vi "Samsung Test Bench.vi"() -> ()   [LabVIEW 2014]
uses:
  Controls/NamedError.ctl
  Controls/ES String Data.ctl
  Controls/ES String Array.ctl
  Controls/StringSelector.ctl
  Controls/ES System Data.ctl
  Controls/Gen Data.ctl
panel:
  out "Generator Fault String":string
  out "Generator Data":T1 {"Alarms" format="%04x"}
  out "PDP Control Error":T2
  in  "PDP Contact On":bool
  in  "Reset Samsung":bool
  in  "Clear Error":bool
  in  "Generator On":bool
  out "Generator Error":T2
  out "Voltage 2":sgl format="%3.0f V"
  out "Voltage 1":sgl format="%3.0f V"
  in  "Contactor 2":bool
  in  "Contactor 1":bool
  out "Battery System Data":T3={"Voltage"=0.0, "Current"=0.0, "SOC Avg"=0.0, "Faults"=0, "Alarms"=0, "# Strings"=0, "Max Temp"=0, "Min Temp"=0, "Max Cell Voltage"=0.0, "Min Cell Voltage"=0.0, "Energy Capacity"=0.0, "Energy Remaining"=0.0, "SOC Min"=0.0, "SOC Max"=0.0, "ES Fault"=FALSE, "String Select"=enum."3 Strings", "ES Com Fault"=FALSE, "SOH Avg"=0.0}
  out "Battery Rack Data":T5
  out "Battery Error":T2
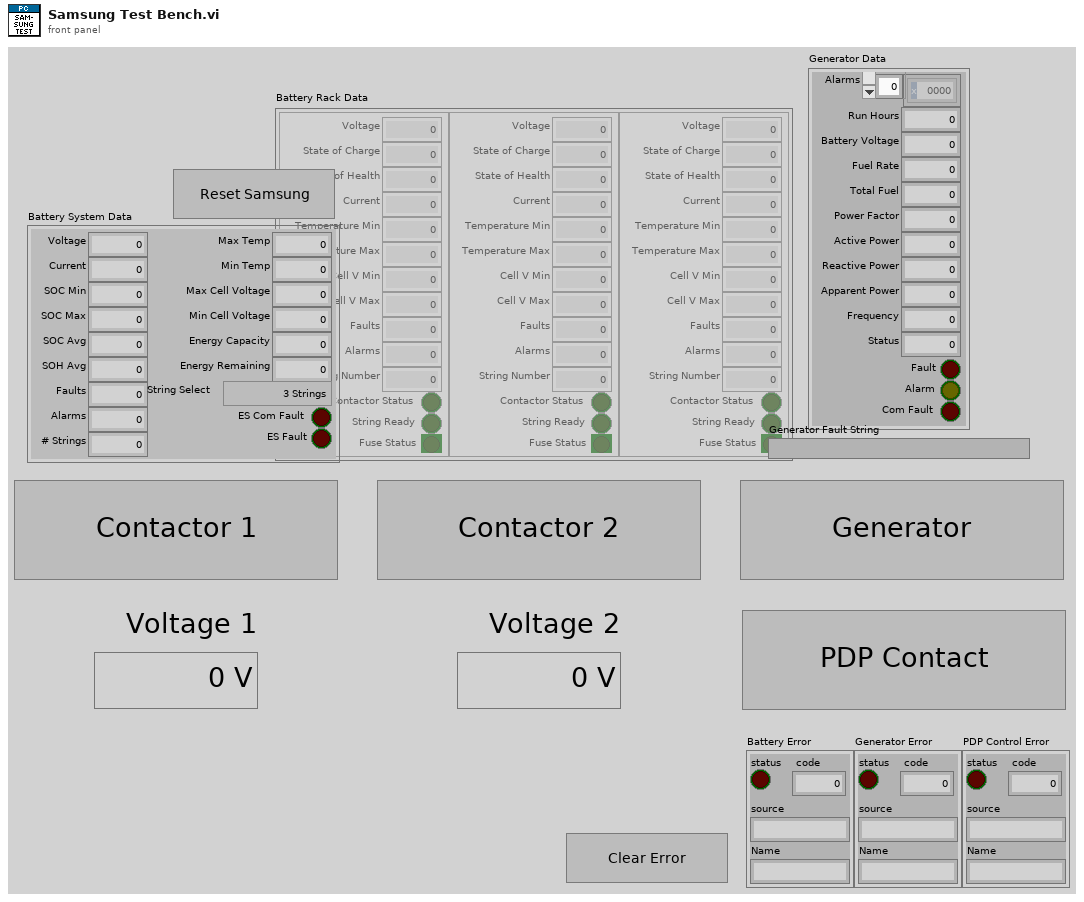
[diagram p1: front panel]
types:
  T1 = typedef "Gen Data.ctl" = cluster{"Alarms":i16[], "Run Hours":dbl, "Battery Voltage":dbl, "Fuel Rate":dbl, "Total Fuel":dbl, "Power Factor":dbl, "Active Power":dbl, "Reactive Power":dbl, "Apparent Power":dbl, "Frequency":dbl, "Status":u16, "Fault":bool, "Alarm":bool, "Com Fault":bool}
  T2 = typedef "NamedError.ctl" = cluster{"status":bool, "code":i32, "source":string, "Name":string}
  T3 = typedef "ES System Data.ctl" = cluster{"Voltage":sgl, "Current":sgl, "SOC Avg":sgl, "Faults":u16, "Alarms":u16, "# Strings":u16, "Max Temp":i16, "Min Temp":i16, "Max Cell Voltage":sgl, "Min Cell Voltage":sgl, "Energy Capacity":sgl, "Energy Remaining":sgl, "SOC Min":sgl, "SOC Max":sgl, "ES Fault":bool, "String Select":T4, "ES Com Fault":bool, "SOH Avg":sgl}
  T4 = typedef "StringSelector.ctl" = enum16{"1 String (1)", "1 String (2)", "1 String (3)", "2 Strings (1 2)", "2 Strings (2 3)", "2 Strings (1 3)", "3 Strings"}
  T5 = typedef "ES String Array.ctl" = T6[]
  T6 = typedef "ES String Data.ctl" = cluster{"Voltage":sgl, "State of Charge":sgl, "Current":sgl, "Temperature Min":i16, "Temperature Max":i16, "Faults":u16, "Alarms":u16, "String Number":u16, "Contactor Status":bool, "String Ready":bool, "Fuse Status":bool, "Cell V Max":dbl, "Cell V Min":dbl, "State of Health":sgl}
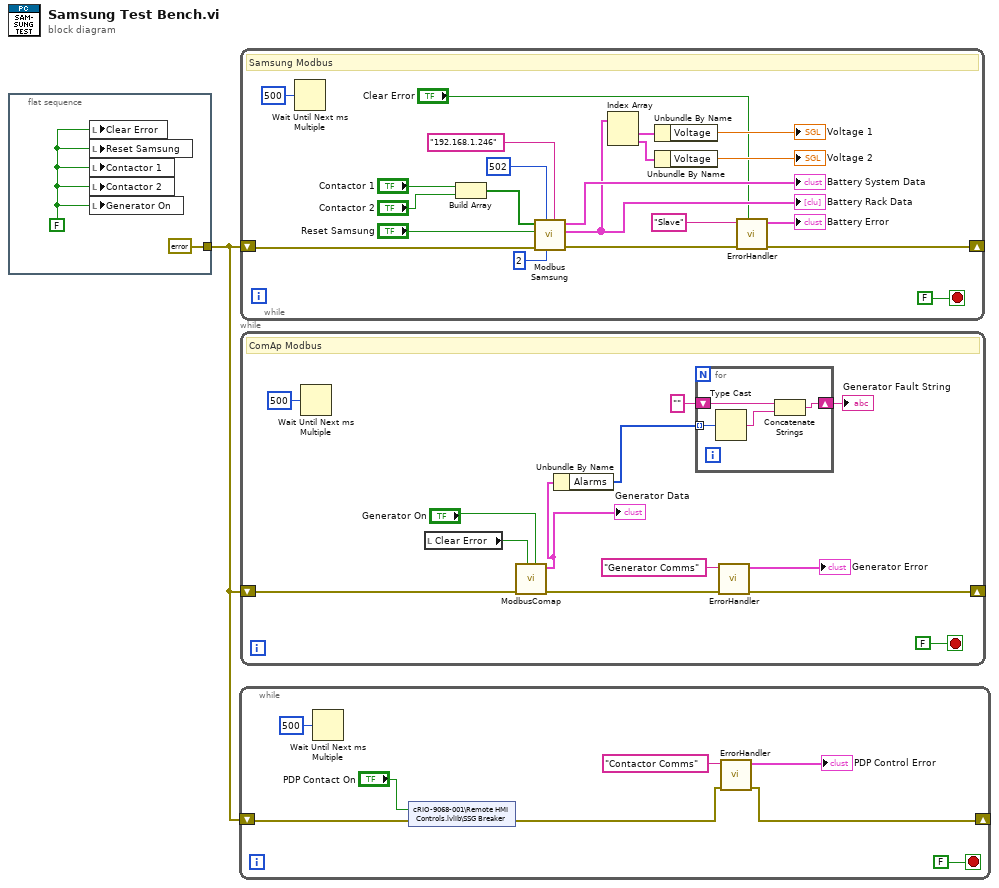
[diagram p0: block diagram]
diagram:
  n1 = flat-sequence {
    tunnel: [errorcluster {"status"=FALSE, "code"=0, "source"=""} ("Error Out")] -> w1
    frame #0 {
      w2 = FALSE ("ES Reset")
      n2 = local write "Clear Error"(w2) -> ()
      n3 = local write "Reset Samsung"(w2) -> ()
      n4 = local write "Contactor 1"(w2) -> ()
      n5 = local write "Contactor 2"(w2) -> ()
      n6 = local write "Generator On"(w2) -> ()
    }
  }
  n7 = while {
    shift-right: [w7] -> _
    shift-left: w1 -> [w11]
    stop <- FALSE stop-if-true
    n8 = Wait Until Next ms Multiple(millisecond multiple=u32 500 ("milliseconds to wait")) -> ()  [unwired: 1 out]
    n9 = shared-variable "cRIO-9068-001\\Remote HMI Controls.lvlib\\SSG Breaker"("PDP Contact On", error in=w11) -> (error out=w8:errorcluster)
    n10 = call "ErrorHandler.vi"("Error In"=w8, "Name"="Contactor Comms") -> ("Error Out"=w7:errorcluster, "Named Error Out"=→"PDP Control Error":T2)  [unwired: 6 in]
  }
  n11 = while {
    shift-right: [w31] -> _
    shift-left: w1 -> [w30]
    stop <- FALSE stop-if-true
    # "Samsung Modbus"
    n12 = Wait Until Next ms Multiple(millisecond multiple=u32 500 ("milliseconds to wait")) -> ()  [unwired: 1 out]
    n13 = Build Array("Contactor 1", "Contactor 2") -> (w19:bool[])
    n14 = call "Modbus Samsung.vi"("address"="192.168.1.246", "# Racks"=u8 2, "port (502)"=u16 502, "Error In"=w30, "ES Reset"="Reset Samsung", "ES ON Array"=w19) -> ("Error Out"=w32:errorcluster, "Energy Storage String Data Out"=w18:T5, "Energy Storage System Data Out"=→"Battery System Data":T3)  [unwired: 1 in, 2 out]
    "Battery Rack Data" <- w18
    n15 = Index Array(array=w18) -> (element #1=w17:T6, element #2=w16:T6)  [unwired: 2 in]
    n16 = Unbundle By Name(w17) -> ("Voltage"=→"Voltage 1":sgl)
    n17 = Unbundle By Name(w16) -> ("Voltage"=→"Voltage 2":sgl)
    n18 = call "ErrorHandler.vi"("Clear Error"="Clear Error", "Error In"=w32, "Name"="Slave") -> ("Error Out"=w31:errorcluster, "Named Error Out"=→"Battery Error":T2)  [unwired: 5 in]
  }
  n19 = while {
    shift-right: [w41] -> _
    shift-left: w1 -> [w37]
    stop <- FALSE stop-if-true
    # "ComAp Modbus"
    n20 = Wait Until Next ms Multiple(millisecond multiple=u32 500 ("milliseconds to wait")) -> ()  [unwired: 1 out]
    n21 = local read "Clear Error"() -> (w38:bool)
    n22 = call "ModbusComap.vi"("Generator On"="Generator On", "Clear Alarms"=w38, "Error In"=w37) -> ("Error Out"=w42:errorcluster, "Gen Data"=w34:T1)  [unwired: 5 in]
    "Generator Data" <- w34
    n23 = Unbundle By Name(w34) -> ("Alarms"=w33:i16[])
    n24 = for {
      tunnel: w33 -> [w49] mode=indexing
      shift-right: [w48] -> w36
      shift-left: "" -> [w46]
      n25 = Type Cast(x=w49) -> (*(type *) &x=w47:string)  [unwired: 1 in]
      n26 = Concatenate Strings(w46, w47) -> (w48:string)
    }
    "Generator Fault String" <- w36
    n27 = call "ErrorHandler.vi"("Error In"=w42, "Name"="Generator Comms") -> ("Error Out"=w41:errorcluster, "Named Error Out"=→"Generator Error":T2)  [unwired: 6 in]
  }
